vi "Get LakeShore 370 Resistance.vi"   [LabVIEW 2015]
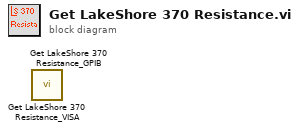
[diagram p0: block diagram]
diagram:
  n1 = call "Get LakeShore 370 Resistance_VISA.vi"() -> ()  [unwired: 9 in, 3 out]
  n2 = call "Get LakeShore 370 Resistance_GPIB.vi"() -> ()  [unwired: 10 in, 2 out]
